vi "Exemple_Preprocessing_MinMaxScaler.vi"() -> ()   [LabVIEW 2020]
uses:
  Objet/6 - Datasets Transformation/6.3 - Processing Data/MinMaxScaler/MinMaxScaler.lvclass
panel:
  in  "X":string[][](array[string])=[["-1", "2"], ["-0,5", "6"], ["0", "10"], ["1", "18"]]
  in  "y":string[][](array[string])
  out "Data":T1
  out "error out":errorcluster
  in  "error in":errorcluster caption="entrée d'erreur"
  in  "MinMaxScaler":T2={"feature_range"={"min"=0.0, "max"=1.0}, "copy"=TRUE}
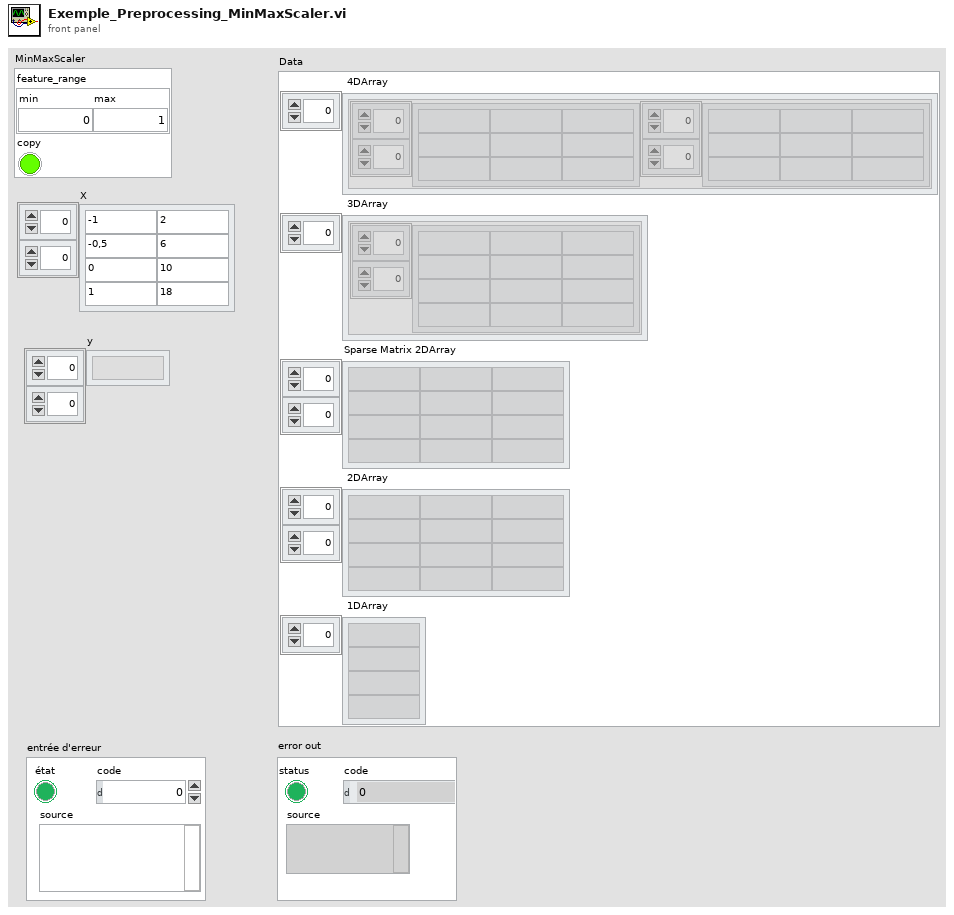
[diagram p1: front panel]
types:
  T1 = cluster{" 4DArray":cluster{"1":string[][], "2":string[][]}[], " 3DArray":cluster{"Tableau":string[][]}[], "Sparse Matrix 2DArray":string[][], " 2DArray":string[][], " 1DArray":string[]}
  T2 = cluster{"feature_range":cluster{"min":dbl, "max":dbl}, "copy":bool}
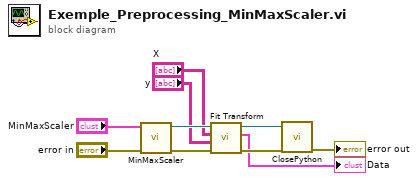
[diagram p0: block diagram]
diagram:
  n1 = call "MinMaxScaler.vi"("error in (no error)"="error in", "MinMaxScaler"="MinMaxScaler") -> ("error out"=w7:errorcluster, "MinMaxScaler.lvclass"=w8:refnum<class "MinMaxScaler.lvclass">)  [unwired: 8 in]
  n2 = call-dynamic "Fit Transform.vi"("error in (no error)"=w7, "y"="y", "X"="X", "MinMaxScaler.lvclass"=w8) -> ("error out"=w5:errorcluster, "Data"=→"Data":T1, "MinMaxScaler.lvclass"=w6:refnum<class "MinMaxScaler.lvclass">)  [unwired: 5 in]
  n3 = call-dynamic "ClosePython.vi"("error in (no error)"=w5, "Scikit-learn en entrée"=w6) -> ("error out"=→"error out":errorcluster)  [unwired: 8 in, 1 out]
